vi "Periodic Tasks.vi"() -> ()   [LabVIEW 2011]
doc: "This VI runs in parallel to other tasks. It can contain as many user-defined periodic loops as you need. These can carry out PID or other sorts of timed response."
uses:
  <vilib>/Rock Robotics/SystemInterfaces/Utilities/FPGA_UtilitiesLED State.ctl
  <vilib>/Rock Robotics/SystemInterfaces/Utilities/FPGA_UtilitiesLED Source.ctl
  <vilib>/Rock Robotics/WPI/Relay/WPI_RelayValue.ctl
  Robot Global Data.vi
panel:
  in  "Dial Shooter Calibration Min Volt":dbl
  in  "Dial Shooter Calibration Max Volt":dbl=3.3
  out "Sent?":string="File Wrote"
  out "Voltage":dbl
  in  "Recording Array":dbl[][](array[numeric])
  in  "Turn on Record 2":bool
  out "Auton Recording 2":bool
  in  "Home Speed 2":dbl=1.0
  out "Ramp ACT Pot 2":dbl
  out "Auton Recording":bool
  in  "Turn on Record":bool
  in  "Auton Array":dbl[][](array[numeric])
  out "Right Rate":dbl
  out "Right Direction":bool
  out "Right Distance":dbl
  out "Shooter Encoder Distance":dbl
  out "Shooter Direction":bool
  out "Shooter Encoder Rate":dbl
  out "Left Rate":dbl
  out "Gyro Rate":dbl
  out "Gyro Angle":dbl
  out "Left Direction":bool
  out "Left Distance":dbl
  # "Auton Recording"
  # "Sensor Feedback"
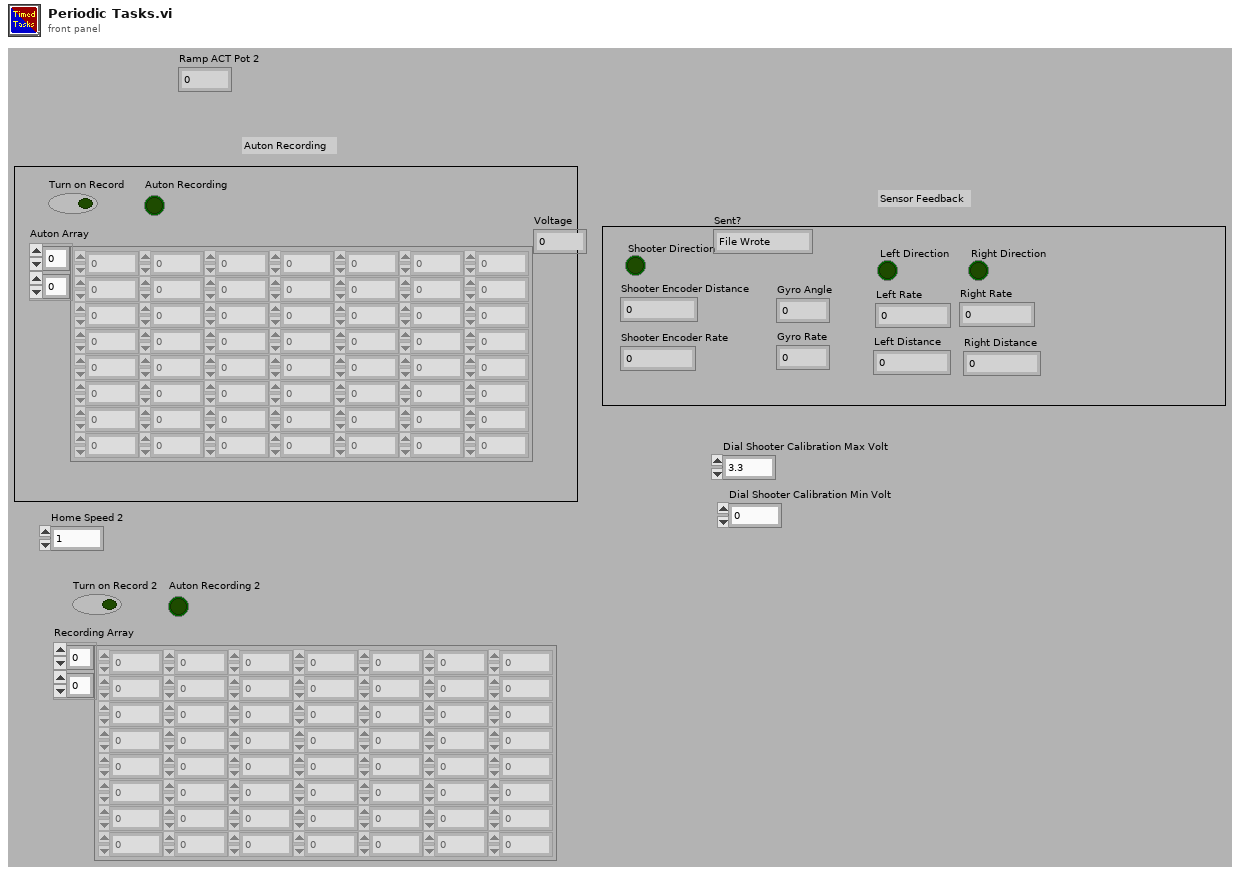
[diagram p1: front panel]
types:
  T1 = typedef "WPI_RelayValue.ctl" = enum16{"Off", "On", "Forward", "Reverse"}
  T2 = cluster{"Driver Station Digital Input (1-8)[0]":bool, "Driver Station Digital Input (1-8)[1]":bool, "Driver Station Digital Input (1-8)[2]":bool, "Driver Station Digital Input (1-8)[3]":bool, "Driver Station Digital Input (1-8)[4]":bool, "Driver Station Digital Input (1-8)[5]":bool, "Driver Station Digital Input (1-8)[6]":bool, "Driver Station Digital Input (1-8)[7]":bool, "Driver Station Digital Input (1-8)[8]":bool}
  T3 = typedef "WPI_AnalogChannelDevRef.ctl" = cluster{"DevStatus":errorcluster, "Analog Module":T4, "Analog Channel":T5}
  T4 = typedef "FPGA_TypedefAnalogModule.ctl" = enum16{"Analog Module 1", "Analog Module 2"}
  T5 = typedef "FPGA_AIChannel.ctl" = enum8{"AI 1", "AI 2", "AI 3", "AI 4", "AI 5", "AI 6", "AI 7", "AI 8", "Invalid"}
  T6 = typedef "WPI_EncoderDevRef.ctl" = cluster{"DevStatus":errorcluster, "EncoderIndex":T7, "CounterIndex":T8, "DistancePerCount":dbl, "Decoding Type":T9}
  T7 = typedef "FPGA_EncoderIdx.ctl" = enum8{"Enc 0", "Enc 1", "Enc 2", "Enc 3", "Invalid"}
  T8 = typedef "FPGA_CounterCtrSystemIndex.ctl" = enum8{"Ctr 0", "Ctr 1", "Ctr 2", "Ctr 3", "Ctr 4", "Ctr 5", "Ctr 6", "Ctr 7", "Invalid"}
  T9 = typedef "WPI_EncoderType.ctl" = enum16{"1x", "2x", "4x"}
  T10 = typedef "WPI_GyroDevRef.ctl" = cluster{"DevStatus":errorcluster, "Analog Module":T4, "Analog Channel":T5, "Offset":dbl, "Gain (VoltsPerDegree/Second)":dbl}
  T11 = cluster{"Analog 1 (V)":dbl, "Analog 2 (V)":dbl, "Analog 3 (V)":dbl, "Analog 4 (V)":dbl, "Analog 5 (V)":dbl, "Analog 6 (V)":dbl, "Analog 7 (V)":dbl, "Analog 8 (V)":dbl}
  T12 = typedef "WPI_RelayDevRef.ctl" = cluster{"DevStatus":errorcluster, "Relay Channel":T13, "Digital Module":T14, "Relay Direction":T15}
  T13 = typedef "FPGA_DIORelayChannel.ctl" = enum8{"Relay 1", "Relay 2", "Relay 3", "Relay 4", "Relay 5", "Relay 6", "Relay 7", "Relay 8", "Invalid"}
  T14 = typedef "FPGA_TypedefDigitalModule.ctl" = enum16{"Digital Module 1", "Digital Module 2"}
  T15 = typedef "WPI_RelayDirection.ctl" = enum16{"Both directions", "Forward only", "Reverse only"}
  T16 = typedef "FPGA_UtilitiesLED State.ctl" = enum16{"Off", "On", "Toggle"}
  T17 = typedef "FPGA_UtilitiesLED Source.ctl" = enum16{"User LED", "FPGA LED"}
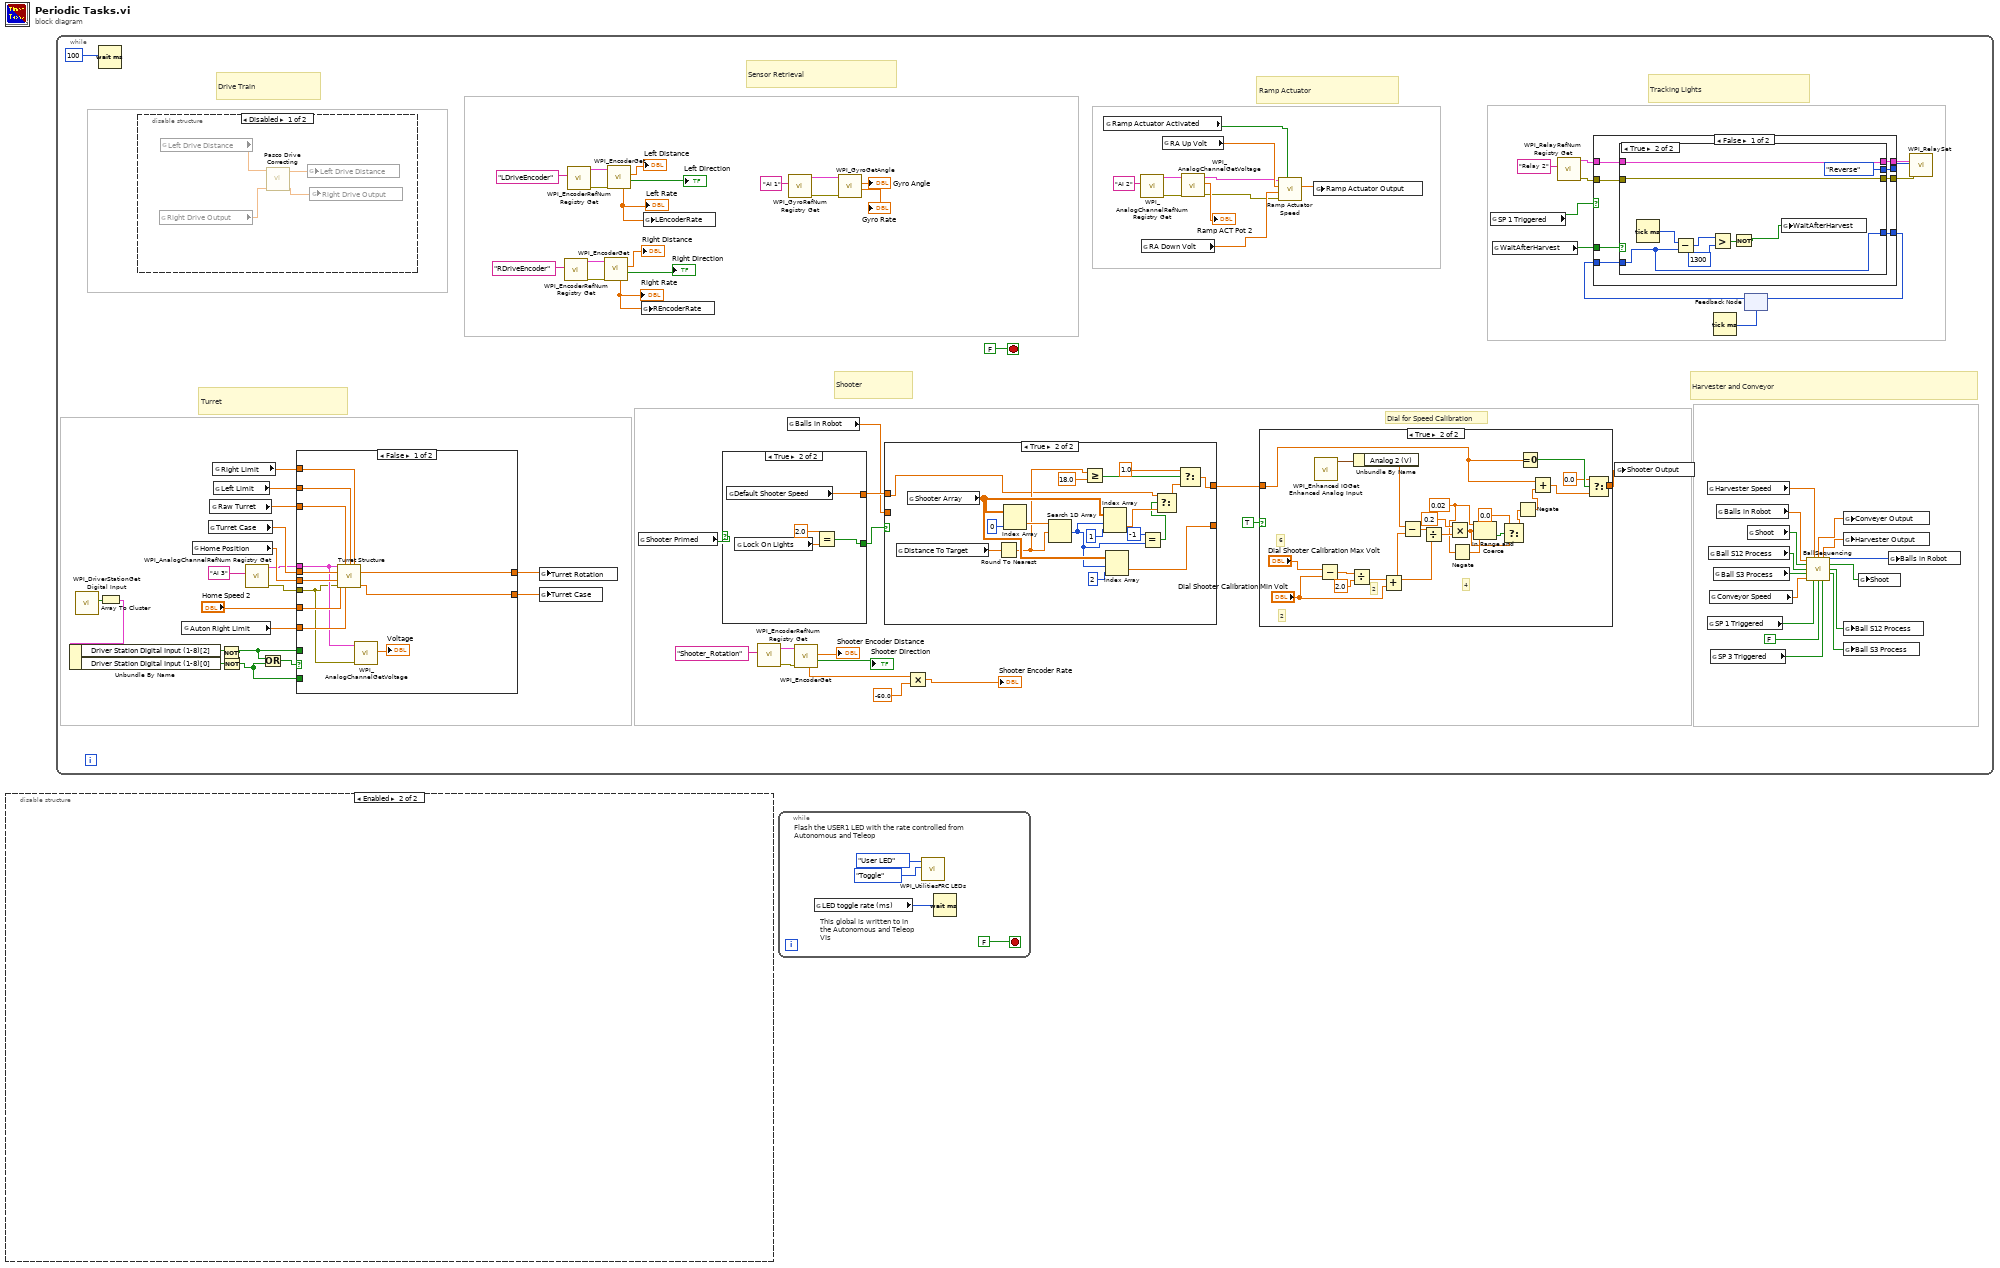
[diagram p0: block diagram]
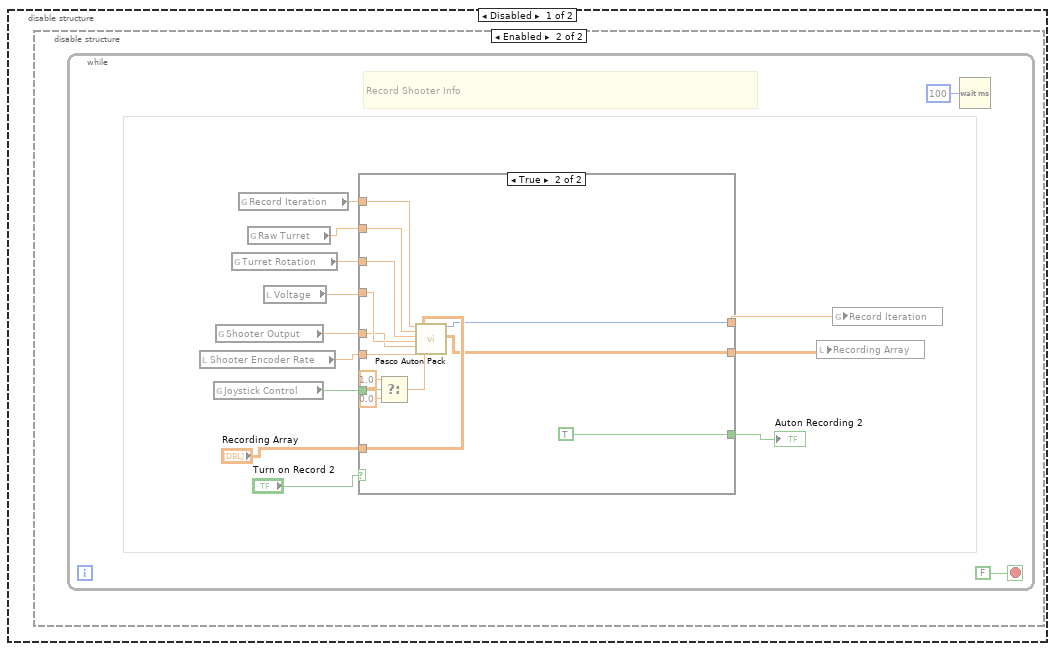
[diagram p2: hidden frame]
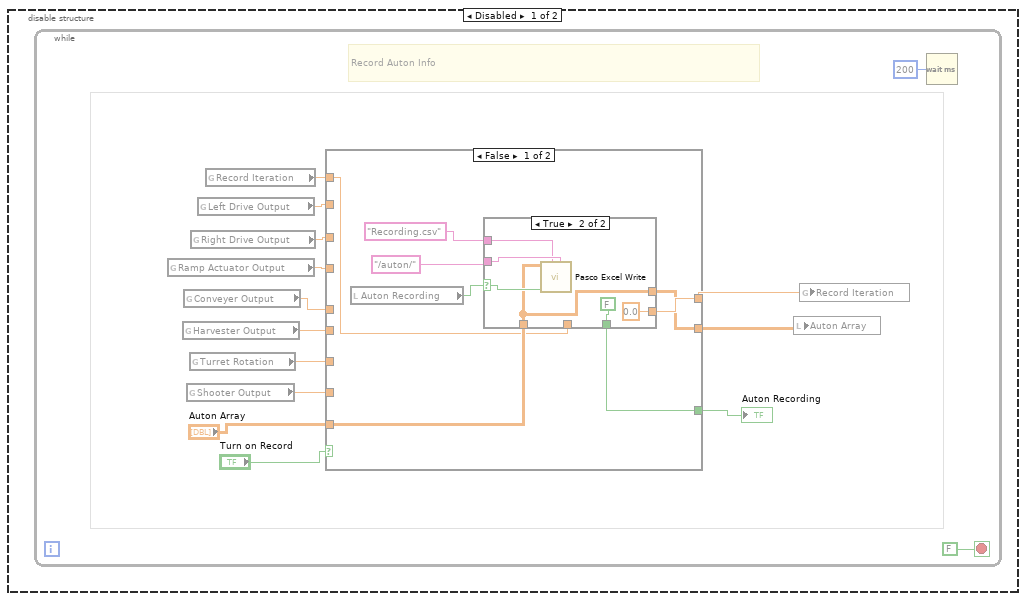
[diagram p3: hidden frame]
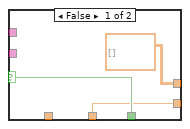
[diagram p4: hidden frame]
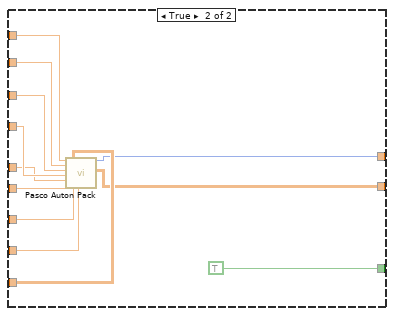
[diagram p5: hidden frame]
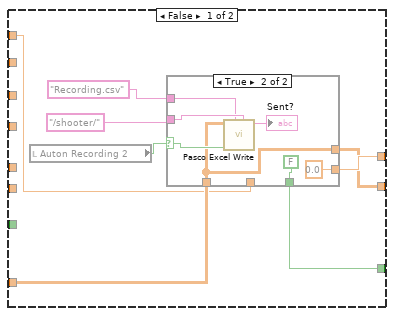
[diagram p6: hidden frame]
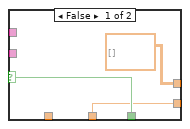
[diagram p7: hidden frame]
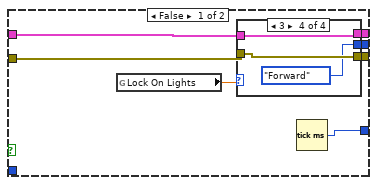
[diagram p9: hidden frame]
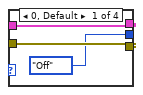
[diagram p10: hidden frame]
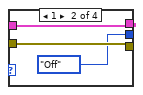
[diagram p11: hidden frame]
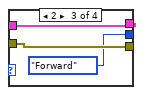
[diagram p12: hidden frame]
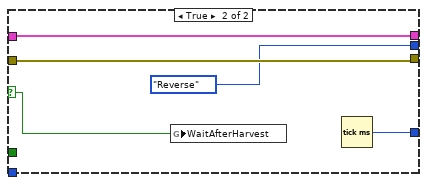
[diagram p13: hidden frame]
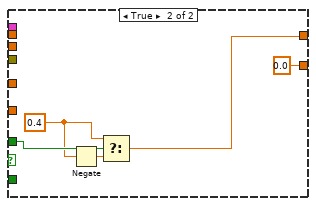
[diagram p14: hidden frame]
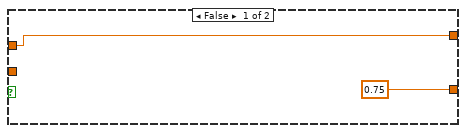
[diagram p15: hidden frame]
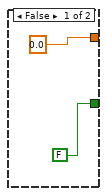
[diagram p16: hidden frame]
diagram:
  n1 = disable-structure shown="Enabled" {
    frame Disabled {
      n2 = disable-structure shown="Enabled" {
        frame Disabled {
          n3 = while {
            stop <- FALSE stop-if-true
            # "Record Auton Info"
            n4 = global read "Robot Global Data.vi" "Ramp Actuator Output"() -> (w5:dbl)
            n5 = global read "Robot Global Data.vi" "Harvester Output"() -> (w7:dbl)
            n6 = global read "Robot Global Data.vi" "Conveyer Output"() -> (w6:dbl)
            n7 = global read "Robot Global Data.vi" "Shooter Output"() -> (w9:dbl)
            n8 = global read "Robot Global Data.vi" "Turret Rotation"() -> (w8:dbl)
            n9 = global read "Robot Global Data.vi" "Right Drive Output"() -> (w4:dbl)
            n10 = global read "Robot Global Data.vi" "Left Drive Output"() -> (w3:dbl)
            n11 = global read "Robot Global Data.vi" "Record Iteration"() -> (w2:dbl)
            n12 = case shown="False" "Turn on Record" {
              tunnel: w2 -> [w19 w44]
              tunnel: w3 -> [_ w43]
              tunnel: w4 -> [_ w42]
              tunnel: w5 -> [_ w41]
              tunnel: w6 -> [_ w40]
              tunnel: w7 -> [_ w39]
              tunnel: w8 -> [_ w38]
              tunnel: w9 -> [_ w37]
              tunnel: "Auton Array" -> [w20 w36]
              tunnel: [w16 w35] -> w12
              tunnel: [w17 w34] -> w13
              tunnel: [w18 TRUE] -> w14
              frame False {
                n13 = local read "Auton Recording"() -> (w21:bool)
                n14 = case shown="True" w21 {
                  selector: w21 -> [w26 w31]
                  tunnel: [w26 FALSE] -> w18
                  tunnel: "/auton/" ("File Name") -> [_ w30]
                  tunnel: "Recording.csv" ("Folder Location") -> [_ w29]
                  tunnel: [w25 0.0 ("Record Iteration")] -> w17
                  tunnel: w19 -> [w25 _]
                  tunnel: w20 -> [_ w27]
                  tunnel: [dbl[][] [] ("Auton Array") w27] -> w16
                  frame False {
                  }
                  frame True {
                    n15 = call "Pasco Excel Write.vi"("Folder Location"=w30, "File Name"=w29, "WriteToExcel"=w31, "2D data"=w27) -> ()  [unwired: 7 in, 1 out]
                  }
                }
              }
              frame True {
                n16 = call "Pasco Auton Pack.vi"("Iterations"=w44, "Left Drive"=w43, "Right Drive"=w42, "RAMP ACT"=w41, "Conveyor"=w40, "Harvestor"=w39, "Auton Array"=w36, "Turret"=w38, "Shooter"=w37) -> ("Iteration Output"=w34:i32, "output array"=w35:dbl[][])  [unwired: 9 in]
              }
            }
            "Auton Recording" <- w14
            n17 = local write "Auton Array"(w12) -> ()
            n18 = global write "Robot Global Data.vi" "Record Iteration"(w13) -> ()
            n19 = Wait (ms)(milliseconds to wait=u32 200) -> ()  [unwired: 1 out]
          }
        }
        frame Enabled {
          n20 = while {
            stop <- FALSE stop-if-true
            # "Record Shooter Info"
            n21 = local read "Shooter Encoder Rate"() -> (w46:dbl)
            n22 = global read "Robot Global Data.vi" "Joystick Control"() -> (w45:bool)
            n23 = global read "Robot Global Data.vi" "Shooter Output"() -> (w47:dbl)
            n24 = global read "Robot Global Data.vi" "Turret Rotation"() -> (w49:dbl)
            n25 = global read "Robot Global Data.vi" "Record Iteration"() -> (w52:dbl)
            n26 = global read "Robot Global Data.vi" "Raw Turret"() -> (w50:dbl)
            n27 = local read "Voltage"() -> (w48:dbl)
            n28 = case shown="True" "Turn on Record 2" {
              tunnel: w52 -> [w62 w90]
              tunnel: w50 -> [_ w89]
              tunnel: w49 -> [_ w88]
              tunnel: w48 -> [_ w87]
              tunnel: w47 -> [_ w86]
              tunnel: w46 -> [_ w85]
              tunnel: "Recording Array" -> [w63 w84]
              tunnel: [w59 w83] -> w55
              tunnel: [w60 w82] -> w56
              tunnel: [w61 TRUE] -> w57
              tunnel: w45 -> [_ w80]
              frame False {
                n29 = local read "Auton Recording 2"() -> (w64:bool)
                n30 = case shown="True" w64 {
                  selector: w64 -> [w69 w75]
                  tunnel: [w69 FALSE] -> w61
                  tunnel: "/shooter/" ("File Name") -> [_ w74]
                  tunnel: "Recording.csv" ("Folder Location") -> [_ w73]
                  tunnel: [w68 0.0 ("Record Iteration")] -> w60
                  tunnel: w62 -> [w68 _]
                  tunnel: w63 -> [_ w71]
                  tunnel: [dbl[][] [] ("Auton Array") w71] -> w59
                  frame False {
                  }
                  frame True {
                    n31 = call "Pasco Excel Write.vi"("Folder Location"=w74, "File Name"=w73, "WriteToExcel"=w75, "2D data"=w71) -> ("Sent?"=→"Sent?":string)  [unwired: 7 in]
                  }
                }
              }
              frame True {
                n32 = Select(t=1.0, s=w80, f=0.0) -> (s? t:f=w77:dbl)
                n33 = call "Pasco Auton Pack.vi"("Iterations"=w90, "Left Drive"=w89, "Right Drive"=w88, "RAMP ACT"=w87, "Conveyor"=w86, "Harvestor"=w85, "Auton Array"=w84, "Turret"=w77) -> ("Iteration Output"=w82:i32, "output array"=w83:dbl[][])  [unwired: 10 in]
              }
            }
            "Auton Recording 2" <- w57
            n34 = local write "Recording Array"(w55) -> ()
            n35 = global write "Robot Global Data.vi" "Record Iteration"(w56) -> ()
            n36 = Wait (ms)(milliseconds to wait=u32 100) -> ()  [unwired: 1 out]
          }
        }
      }
    }
    frame Enabled {
    }
  }
  n37 = while {
    stop <- FALSE stop-if-true
    # "Dial for Speed Calibration"
    # "Tracking Lights"
    # "Harvester and Conveyor"
    # "Shooter"
    # "Sensor Retrieval"
    # "Turret"
    # "Drive Train"
    # "Ramp Actuator"
    n38 = call <vilib>:"WPI_DriverStationGet Digital Input.vi"() -> ("Driver Station Digital Input (1-8)"=w123:bool[])  [unwired: 11 in]
    n39 = Wait (ms)(milliseconds to wait=u32 100) -> ()  [unwired: 1 out]
    n40 = Array To Cluster(array=w123) -> (cluster=w122:T2)
    n41 = Unbundle By Name(w122) -> ("Driver Station Digital Input (1-8)[2]"=w108:bool, "Driver Station Digital Input (1-8)[0]"=w106:bool)
    n42 = disable-structure shown="Disabled" {
      frame Disabled {
        n43 = global read "Robot Global Data.vi" "Right Drive Output"() -> (w290:dbl)
        n44 = global read "Robot Global Data.vi" "Left Drive Distance"() -> (w291:dbl)
        n45 = call "Pasco Drive Correcting.vi"("RightDriveOutput"=w290, "LeftDriveOutput"=w291) -> ("RightDriveOutput"=w288:dbl, "LeftDriveOutput"=w289:dbl)  [unwired: 8 in]
        n46 = global write "Robot Global Data.vi" "Left Drive Distance"(w289) -> ()
        n47 = global write "Robot Global Data.vi" "Right Drive Output"(w288) -> ()
      }
      frame Enabled {
      }
    }
    n48 = global read "Robot Global Data.vi" "Auton Right Limit"() -> (w119:dbl)
    n49 = global read "Robot Global Data.vi" "Home Position"() -> (w114:dbl)
    n50 = global read "Robot Global Data.vi" "Turret Case"() -> (w113:dbl)
    n51 = global read "Robot Global Data.vi" "Raw Turret"() -> (w115:dbl)
    n52 = global read "Robot Global Data.vi" "Right Limit"() -> (w118:dbl)
    n53 = global read "Robot Global Data.vi" "Left Limit"() -> (w117:dbl)
    n54 = Not(x=w108) -> (.not. x?=w107:bool)
    n55 = Not(x=w106) -> (.not. x?=w105:bool)
    n56 = call <vilib>:"WPI_AnalogChannelRefNum Registry Get.vi"("refnum name"="AI 3") -> ("error out"=w112:errorcluster, "AIDeviceRef"=w111:T3)  [unwired: 9 in]
    n57 = Or(x=w107, y=w105) -> (x .or. y?=w109:bool)
    n58 = case shown="False" w109 {
      tunnel: w111 -> [w247 _]
      tunnel: w112 -> [w246 _]
      tunnel: w113 -> [w256 _]
      tunnel: w114 -> [w255 _]
      tunnel: w115 -> [w254 _]
      tunnel: "Home Speed 2" -> [w253 _]
      tunnel: w117 -> [w252 _]
      tunnel: w118 -> [w251 _]
      tunnel: w119 -> [w250 _]
      tunnel: [w249 w260] -> w120
      tunnel: [w248 0.0 ("Turret Case Output")] -> w121
      tunnel: w107 -> [_ w261]
      tunnel: w105 -> [_ _]
      frame False {
        n59 = call "Turret Structure.vi"("AIDeviceRef"=w247, "Raw Turret"=w254, "Left"=w252, "Right"=w251, "Turret Case"=w256, "Home Speed"=w253, "Home postion"=w255, "error in (no error)"=w246, "Auton Right"=w250) -> ("Turret Output"=w249:dbl, "Turret Case Output"=w248:dbl)  [unwired: 5 in]
        n60 = call <vilib>:"WPI_AnalogChannelGetVoltage.vi"("error in (no error)"=w246, "AIDeviceRef"=w247) -> ("Voltage"=→"Voltage":dbl)  [unwired: 7 in, 2 out]
      }
      frame True {
        w257 = 0.4 ("t")
        n61 = Negate(x=w257) -> (-x=w258:dbl)
        n62 = Select(t=w257, s=w261, f=w258) -> (s? t:f=w260:dbl)
      }
    }
    n63 = global write "Robot Global Data.vi" "Turret Rotation"(w120) -> ()
    n64 = global write "Robot Global Data.vi" "Turret Case"(w121) -> ()
    n65 = call <vilib>:"WPI_EncoderRefNum Registry Get.vi"("refnum name"="RDriveEncoder") -> ("error out"=w147:errorcluster, "EncoderDevRef"=w146:T6)  [unwired: 9 in]
    n66 = call <vilib>:"WPI_EncoderRefNum Registry Get.vi"("refnum name"="LDriveEncoder") -> ("error out"=w153:errorcluster, "EncoderDevRef"=w152:T6)  [unwired: 9 in]
    n67 = call <vilib>:"WPI_EncoderGet.vi"("error in (no error)"=w147, "EncoderDevRef"=w146) -> ("Direction"=→"Right Direction":bool, "Distance"=→"Right Distance":dbl, "Rate"=w143:dbl)  [unwired: 4 in, 3 out]
    "Right Rate" <- w143
    n68 = call <vilib>:"WPI_EncoderGet.vi"("error in (no error)"=w153, "EncoderDevRef"=w152) -> ("Direction"=→"Left Direction":bool, "Distance"=→"Left Distance":dbl, "Rate"=w149:dbl)  [unwired: 4 in, 3 out]
    "Left Rate" <- w149
    n69 = global read "Robot Global Data.vi" "Shooter Primed"() -> (w166:bool)
    n70 = global write "Robot Global Data.vi" "REncoderRate"(w143) -> ()
    n71 = global write "Robot Global Data.vi" "LEncoderRate"(w149) -> ()
    n72 = case shown="True" w166 {
      tunnel: [FALSE ("Shooter Primed") w284] -> w125
      tunnel: [0.0 w285] -> w165
      frame False {
      }
      frame True {
        n73 = global read "Robot Global Data.vi" "Default Shooter Speed"() -> (w285:dbl)
        n74 = global read "Robot Global Data.vi" "Lock On Lights"() -> (w287:dbl)
        n75 = Equal?(x=2.0, y=w287) -> (x = y?=w284:bool)
      }
    }
    n76 = call <vilib>:"WPI_EncoderRefNum Registry Get.vi"("refnum name"="Shooter_Rotation") -> ("error out"=w127:errorcluster, "EncoderDevRef"=w128:T6)  [unwired: 9 in]
    n77 = global read "Robot Global Data.vi" "Balls in Robot"() -> (w164:dbl)
    n78 = call <vilib>:"WPI_GyroRefNum Registry Get.vi"("refnum name"="AI 1") -> ("error out"=w161:errorcluster, "GyroDevRef"=w162:T10)  [unwired: 9 in]
    n79 = call <vilib>:"WPI_EncoderGet.vi"("error in (no error)"=w127, "EncoderDevRef"=w128) -> ("Direction"=→"Shooter Direction":bool, "Distance"=→"Shooter Encoder Distance":dbl, "Rate"=w124:dbl)  [unwired: 4 in, 3 out]
    n80 = call <vilib>:"WPI_GyroGetAngle.vi"("error in (no error)"=w161, "GyroDevRef"=w162) -> ("Angular Rate"=→"Gyro Rate":dbl, "Angle"=→"Gyro Angle":dbl)  [unwired: 6 in, 2 out]
    n81 = case shown="True" w125 {
      tunnel: [w263 w272] -> w91
      tunnel: w165 -> [w263 w264]
      tunnel: w164 -> [_ _]
      tunnel: [0.75 w281] -> _
      frame False {
      }
      frame True {
        n82 = global read "Robot Global Data.vi" "Distance To Target"() -> (w278:dbl)
        n83 = global read "Robot Global Data.vi" "Shooter Array"() -> (w275:dbl[][])
        n84 = Round To Nearest(number=w278) -> (nearest integer value=w273:dbl)
        n85 = Index Array(array=w275, index (col)=0 ("disabled index (col)")) -> (element=w277:dbl[])  [unwired: 1 in]
        n86 = Search 1D Array(1D array=w277, element=w273) -> (index of element=w267:i32)  [unwired: 1 in]
        n87 = Greater Or Equal?(x=w273, y=18.0) -> (x >= y?=w271:bool)
        n88 = Index Array(array=w275, index (row)=w267, index (col)=1 ("disabled index (col)")) -> (element=w268:dbl)
        n89 = Index Array(array=w275, index (row)=w267, index (col)=2 ("disabled index (col)")) -> (element=w281:dbl)
        n90 = Equal?(x=-1, y=w267) -> (x = y?=w265:bool)
        n91 = Select(t=w264, s=w265, f=w268) -> (s? t:f=w269:dbl)
        n92 = Select(t=1.0, s=w271, f=w269) -> (s? t:f=w272:dbl)
      }
    }
    n93 = Multiply(x=w124, y=-60.0) -> (x*y=→"Shooter Encoder Rate":dbl)
    n94 = global read "Robot Global Data.vi" "Ramp Actuator Activated"() -> (w138:bool)
    n95 = call <vilib>:"WPI_AnalogChannelRefNum Registry Get.vi"("refnum name"="AI 2") -> ("error out"=w136:errorcluster, "AIDeviceRef"=w137:T3)  [unwired: 9 in]
    n96 = global read "Robot Global Data.vi" "RA Down Volt"() -> (w141:dbl)
    n97 = global read "Robot Global Data.vi" "RA Up Volt"() -> (w140:dbl)
    n98 = call <vilib>:"WPI_AnalogChannelGetVoltage.vi"("error in (no error)"=w136, "AIDeviceRef"=w137) -> ("error out"=w133:errorcluster, "Voltage"=→"Ramp ACT Pot 2":dbl, "AIDeviceRef"=w134:T3)  [unwired: 7 in]
    n99 = case shown="True" TRUE {
      tunnel: [w180 w181] -> w92
      tunnel: w91 -> [w180 w185]
      frame False {
      }
      frame True {
        w191 = 0.02
        # "2"
        # "4"
        # "2"
        # "6"
        n100 = call <vilib>:"WPI_Enhanced IOGet Enhanced Analog Input.vi"() -> ("Analogs (V)"=w203:T11)  [unwired: 9 in, 2 out]
        n101 = Subtract(x="Dial Shooter Calibration Max Volt", y="Dial Shooter Calibration Min Volt") -> (x-y=w201:dbl)
        n102 = Divide(x=w201, y=2.0) -> (x/y=w195:dbl)
        n103 = Unbundle By Name(w203) -> ("Analog 2 (V)"=w198:dbl)
        n104 = Add(x=w195, y="Dial Shooter Calibration Min Volt") -> (x+y=w197:dbl)
        n105 = Subtract(x=w198, y=w197) -> (x-y=w196:dbl)
        n106 = Divide(x=w196, y=w195) -> (x/y=w194:dbl)
        n107 = Multiply(x=0.2, y=w194) -> (x*y=w188:dbl)
        n108 = Negate(x=w191) -> (-x=w192:dbl)
        n109 = In Range and Coerce(upper limit=w191, x=w188, lower limit=w192) -> (In Range?=w190:bool)  [unwired: 1 out]
        n110 = Select(t=0.0, s=w190, f=w188) -> (s? t:f=w187:dbl)
        n111 = Negate(x=w187) -> (-x=w186:dbl)
        n112 = Equal To 0?(x=w185) -> (x = 0?=w184:bool)
        n113 = Add(x=w185, y=w186) -> (x+y=w183:dbl)
        n114 = Select(t=0.0, s=w184, f=w183) -> (s? t:f=w181:dbl)
      }
    }
    n115 = call "Ramp Actuator Speed.vi"("Up to Down"=w138, "error in (no error)"=w133, "RA Down Volt"=w141, "RA Up Volt"=w140, "AIDeviceRef"=w134) -> ("Ramp Actuator Ouput"=w139:dbl)  [unwired: 6 in]
    n116 = global write "Robot Global Data.vi" "Ramp Actuator Output"(w139) -> ()
    n117 = global read "Robot Global Data.vi" "SP 1 Triggered"() -> (w104:bool)
    n118 = global read "Robot Global Data.vi" "WaitAfterHarvest"() -> (w97:bool)
    n119 = call <vilib>:"WPI_RelayRefNum Registry Get.vi"("refnum name"="Relay 2") -> ("error out"=w102:errorcluster, "RelayDevRef"=w100:T12)  [unwired: 9 in]
    n120 = global write "Robot Global Data.vi" "Shooter Output"(w92) -> ()
    n121 = global read "Robot Global Data.vi" "Harvester Speed"() -> (w163:dbl)
    n122 = global read "Robot Global Data.vi" "SP 1 Triggered"() -> (w169:bool)
    n123 = global read "Robot Global Data.vi" "Ball S12 Process"() -> (w171:bool)
    n124 = global read "Robot Global Data.vi" "Conveyor Speed"() -> (w155:dbl)
    n125 = global read "Robot Global Data.vi" "SP 3 Triggered"() -> (w168:bool)
    n126 = Tick Count (ms)() -> (millisecond timer value=w94:u32)
    n127 = global read "Robot Global Data.vi" "Ball S3 Process"() -> (w170:bool)
    n128 = global read "Robot Global Data.vi" "Balls in Robot"() -> (w173:dbl)
    n129 = feedback #1(w94) -> (w95:u32)
    n130 = case shown="False" w104 {
      selector: w104 -> [_ w241]
      tunnel: [w211 w244] -> w99
      tunnel: w100 -> [w210 w244]
      tunnel: [w209 w243] -> w101
      tunnel: w102 -> [w208 w243]
      tunnel: [w207 WPI_RelayValue."Reverse" ("RelayValue")] -> w103
      tunnel: [w204 w240] -> w96
      tunnel: w97 -> [w206 _]
      tunnel: w95 -> [w205 _]
      frame False {
        n131 = case shown="True" w206 {
          tunnel: [w218 w239] -> w211
          tunnel: w210 -> [w217 w239]
          tunnel: [w216 w238] -> w209
          tunnel: w208 -> [w215 w238]
          tunnel: [w214 WPI_RelayValue."Reverse" ("RelayValue")] -> w207
          tunnel: w205 -> [_ w231]
          tunnel: [w212 w231] -> w204
          frame False {
            n132 = global read "Robot Global Data.vi" "Lock On Lights"() -> (w213:dbl)
            n133 = case shown="3" w213 {
              tunnel: [w221 w224 w227 w230] -> w218
              tunnel: w217 -> [w221 w224 w227 w230]
              tunnel: [w220 w223 w226 w229] -> w216
              tunnel: w215 -> [w220 w223 w226 w229]
              tunnel: [WPI_RelayValue."Off" ("RelayValue") WPI_RelayValue."Off" ("RelayValue") WPI_RelayValue."Forward" ("RelayValue") WPI_RelayValue."Forward" ("RelayValue")] -> w214
              frame 0, Default {
              }
              frame 1 {
              }
              frame 2 {
              }
              frame 3 {
              }
            }
            n134 = Tick Count (ms)() -> (millisecond timer value=w212:u32)
          }
          frame True {
            n135 = Tick Count (ms)() -> (millisecond timer value=w236:u32)
            n136 = Subtract(x=w236, y=w231) -> (x-y=w235:u32)
            n137 = Greater?(x=w235, y=u32 1300) -> (0:w233:bool)
            n138 = Not(x=w233) -> (.not. x?=w232:bool)
            n139 = global write "Robot Global Data.vi" "WaitAfterHarvest"(w232) -> ()
          }
        }
      }
      frame True {
        n140 = global write "Robot Global Data.vi" "WaitAfterHarvest"(w241) -> ()
        n141 = Tick Count (ms)() -> (millisecond timer value=w240:u32)
      }
    }
    n142 = feedback-in #1(w96) -> ()
    n143 = global read "Robot Global Data.vi" "Shoot"() -> (w172:bool)
    n144 = call "BallSequencing.vi"("Balls In Robot"=w173, "Speed of Harvester"=w163, "Shoot"=w172, "Ball S12 Process"=w171, "Ball S3 Process"=w170, "Speed of Conveyor"=w155, "SP 1 Triggered"=w169, "SP 2 Triggered"=FALSE, "SP 3 Triggered"=w168) -> ("Conveyer Output"=w174:dbl, "Harvester Output"=w175:dbl, "Balls In Robot Output"=w157:i32, "Shoot Output"=w156:bool, "Ball S12 Process Output"=w177:bool, "Ball S3 Process Output"=w176:bool)  [unwired: 1 in]
    n145 = global write "Robot Global Data.vi" "Conveyer Output"(w174) -> ()
    n146 = global write "Robot Global Data.vi" "Harvester Output"(w175) -> ()
    n147 = global write "Robot Global Data.vi" "Ball S12 Process"(w177) -> ()
    n148 = global write "Robot Global Data.vi" "Ball S3 Process"(w176) -> ()
    n149 = global write "Robot Global Data.vi" "Shoot"(w156) -> ()
    n150 = global write "Robot Global Data.vi" "Balls in Robot"(w157) -> ()
    n151 = call <vilib>:"WPI_RelaySet.vi"("error in (no error)"=w101, "RelayValue"=w103, "RelayDevRef"=w99) -> ()  [unwired: 7 in, 2 out]
  }
  n152 = while {
    stop <- FALSE stop-if-true
    # "This global is written to in the Autonomous and Teleop VIs"
    # "Flash the USER1 LED with the rate controlled from Autonomous and Teleop"
    n153 = global read "Robot Global Data.vi" "LED toggle rate (ms)"() -> (w292:u32)
    n154 = call <vilib>:"WPI_UtilitiesFRC LEDs.vi"("State"=FPGA_UtilitiesLED_State."Toggle", "LED Type"=FPGA_UtilitiesLED_Source."User LED") -> ()  [unwired: 1 in, 9 out]
    n155 = Wait (ms)(milliseconds to wait=w292) -> ()  [unwired: 1 out]
  }
